vi "Read PlatMods.vi"(8 "error in (no error)":errorcluster, 11 "TreeDoubleClickMsg in":refnum<class "TreeDoubleClickMsg.lvclass">) -> (0 "error out":errorcluster, 2 "PlatMods":T1, 3 "TreeDoubleClickMsg out":refnum<class "TreeDoubleClickMsg.lvclass">)   [LabVIEW 2017, in "ActorEvents.lvlib" / "TreeDoubleClickMsg.lvclass"]
uses:
  TreeDoubleClickMsg.lvclass
  TreeDoubleClickMsg.lvclass/TreeDoubleClickMsg.ctl
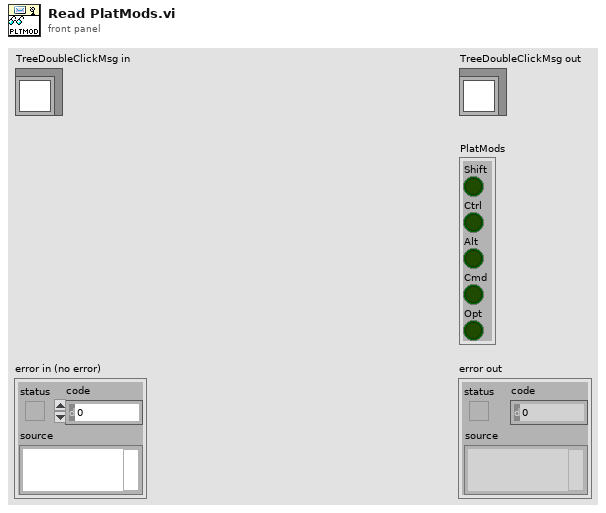
[diagram p1: front panel]
types:
  T1 = cluster{"Shift":bool, "Ctrl":bool, "Alt":bool, "Cmd":bool, "Opt":bool}
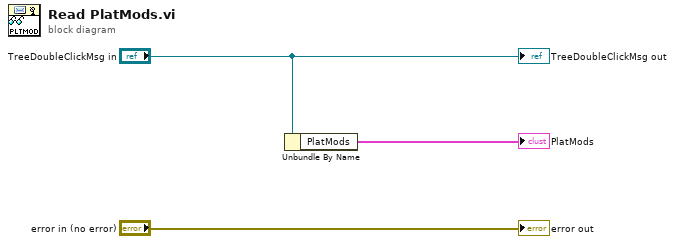
[diagram p0: block diagram]
diagram:
  n1 = Unbundle By Name("TreeDoubleClickMsg in") -> ("PlatMods"=→"PlatMods":T1)
  "error out" <- "error in (no error)"
  "TreeDoubleClickMsg out" <- "TreeDoubleClickMsg in"
